vi "XLP80_HH_Globals.vi"() -> ()   [LabVIEW 2021]
uses:
  XLP80_HH_TDefsCluster_HH Setpoint.ctl
  XLP80_HH_TDefsCluster_HH Feedback.ctl
panel:
  out "Feedback HH":T1 {"Power" format="%.2f W"; "Voltage" format="%.2f V"; "Current" format="%.2f A"}
  in  "Setpoint HH":T2 {"Set Power" min=0 max=64000 step=100 format="%.0f W"; "Set Voltage" format="%.2f V"; "Set Current" format="%.2f A"}
  # "Feedback HH Load"
  # "Set HH Load"
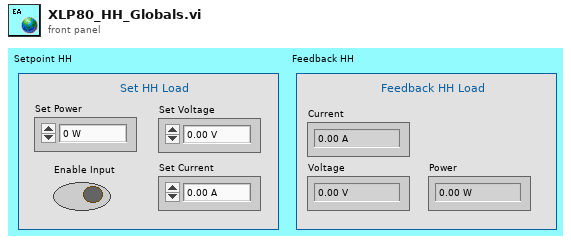
[diagram p1: front panel]
types:
  T1 = typedef "XLP80_HH_TDefsCluster_HH Feedback.ctl" = cluster{"Current":sgl, "Voltage":sgl, "Power":sgl}
  T2 = typedef "XLP80_HH_TDefsCluster_HH Setpoint.ctl" = cluster{"Enable Input":bool, "Set Current":sgl, "Set Voltage":sgl, "Set Power":sgl}
diagram:
